vi "oa_Draw Cursor Labels and Other Indications.vi"(4 "cursor attributes":T2={"layout color"=852223, "active color"=16740820, "precision"=2, "BG transparent? (T)"=TRUE, "radius"=2}, 5 "shaft center line settings":T6={"cartesian grid cosmetics"={"line color"=39168, "text color"=65280, "tick length(3)"=3, "crossing axes"=FALSE, "visible grid?"=TRUE}, "XY plot cosmetics"={"plot color"=16776960, "XY plot type"=enum."connected points", "baseline"=0.0}, "desired font(Application)"=enum."Application Font", "[user-specified font]"={"Font Name:"="", "Size"=0, "Strikeout?"=FALSE, "Italic?"=FALSE, "Underline?"=FALSE, "Outline?"=FALSE, "Shadow?"=FALSE, "Bold?"=FALSE}} {"XY plot cosmetics"."baseline" format="%0.2f"}, 6 "label settings":T3={"show label? (Y)"=TRUE, "avoid overlap? (Y)"=TRUE}, 8 "error in (no error)":errorcluster, 9 "scale info":T1, 10 "Cursor List (EU position]":T4(array[cluster]) {"Location"."phase" format="%.2f"; "Location"."mag" format="%.2f"}, 11 "picture":picture) -> (0 "error out":errorcluster, 3 "new picture":picture)   [LabVIEW 2017]
uses:
  <vilib>/picture/cartesn2.llb/XY Plot Type.ctl
  <vilib>/addons/Sound and Vibration/Order Analysis/Backward Compatibility/SubVIs/OAT Polar Cursor Attributes.ctl
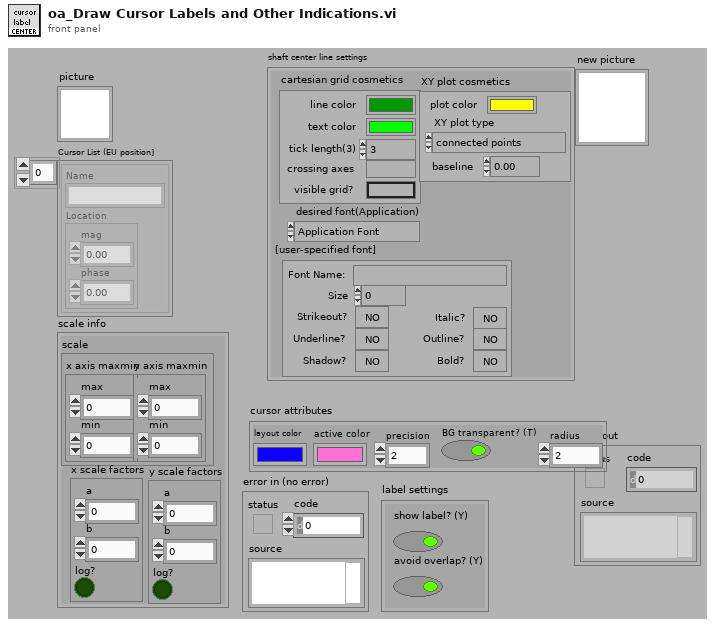
[diagram p1: front panel]
types:
  T1 = cluster{"scale":cluster{"x axis maxmin":cluster{"max":dbl, "min":dbl}, "y axis maxmin":cluster{"max":dbl, "min":dbl}}, "x scale factors":cluster{"a":dbl, "b":dbl, "log?":bool}, "y scale factors":cluster{"a":dbl, "b":dbl, "log?":bool}}
  T2 = typedef "OAT Polar Cursor Attributes.ctl" = cluster{"layout color":u32, "active color":u32, "precision":i16, "BG transparent? (T)":bool, "radius":i16}
  T3 = cluster{"show label? (Y)":bool, "avoid overlap? (Y)":bool}
  T4 = cluster{"Name":string, "Location":cluster{"mag":dbl, "phase":dbl}}[]
  T5 = typedef "XY Plot Type.ctl" = enum16{"points", "squares", "circles", "connected points", "connected squares", "connected circles", "comb plot", "sized scatter plot", "sized-colored scatter plot", "min-max lines"}
  T6 = cluster{"cartesian grid cosmetics":cluster{"line color":u32, "text color":u32, "tick length(3)":i16, "crossing axes":bool, "visible grid?":bool}, "XY plot cosmetics":cluster{"plot color":u32, "XY plot type":T5, "baseline":dbl}, "desired font(Application)":enum16{"User-specified Font", "Application Font", "System Font", "Dialog Font"}, "[user-specified font]":cluster{"Font Name:":string, "Size":i16, "Strikeout?":bool, "Italic?":bool, "Underline?":bool, "Outline?":bool, "Shadow?":bool, "Bold?":bool}}
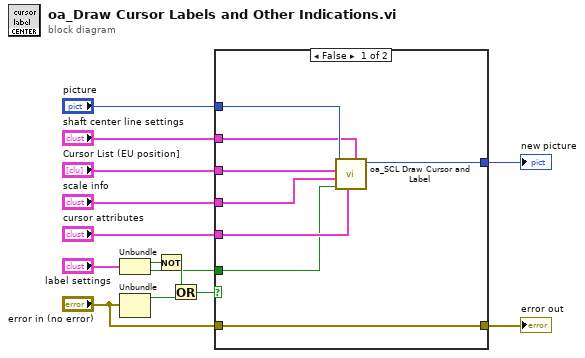
[diagram p0: block diagram]
diagram:
  n1 = Unbundle("label settings") -> ("show label? (Y)"=w6:bool, "avoid overlap? (Y)"=w5:bool)
  n2 = Unbundle("error in (no error)") -> ("status"=w13:bool)  [unwired: 2 out]
  n3 = Not(x=w6) -> (.not. x?=w12:bool)
  n4 = Or(x=w12, y=w13) -> (x .or. y?=w11:bool)
  n5 = case shown="False" w11 {
    tunnel: [w22 w24] -> w10
    tunnel: "error in (no error)" -> [w22 w24]
    tunnel: "picture" -> [w21 w23]
    tunnel: [w17 w23] -> w7
    tunnel: w5 -> [w18 _]
    tunnel: "Cursor List (EU position]" -> [w20 _]
    tunnel: "cursor attributes" -> [w19 _]
    tunnel: "shaft center line settings" -> [w15 _]
    tunnel: "scale info" -> [w16 _]
    frame False {
      n6 = call <vilib>:"oa_SCL Draw Cursor and Label.vi"("shaft center line settings"=w15, "cursor attributes"=w19, "avoid overlap? (Y)"=w18, "scale info"=w16, "Cursor List"=w20, "picture"=w21) -> ("new picture"=w17:picture)  [unwired: 5 in]
    }
    frame True {
    }
  }
  "new picture" <- w7
  "error out" <- w10
